vi "Close.vi"(8 "error in":errorcluster, 11 "Cfg Dev in":refnum<class "Configurable Device.lvclass">) -> (0 "error out":errorcluster, 3 "Cfg Dev out":refnum<class "Configurable Device.lvclass">)   [LabVIEW 2018, in "Configurable Device.lvclass"]
uses:
  Configurable Device.lvclass
  Reusable/Session APIs/File Access/Config Data/Config Data.lvclass
  C:/Program Files (x86)/National Instruments/LabVIEW 2018/vi.lib/MSR Consulting, LLC/General Reuse/Session APIs/_Session Fwk/Session - Root.lvclass
  Configurable Device.lvclass/Configurable Device.ctl
  <vilib>/MSR Consulting, LLC/General Reuse/Session APIs/_Session Fwk/Session - Root.lvclass
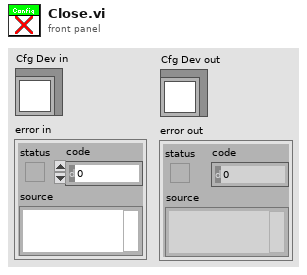
[diagram p1: front panel]
types:
  T1 = typedef "Config Data.lvclass/Config Session.ctl" = refnum<data-value>
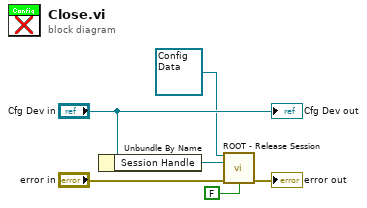
[diagram p0: block diagram]
diagram:
  n1 = Unbundle By Name("Cfg Dev in") -> ("Session Handle"=w4:T1)
  n2 = call <vilib>:"ROOT - Release Session.vi"("OBJ - Session in"=refnum<class "Config Data.lvclass"> refnum ("Config Data"), "Session Handle in"=w4, "error in (no error)"="error in", "force destroy? (F)"=FALSE) -> ("error out"=→"error out":errorcluster)  [unwired: 10 in, 1 out]
  "Cfg Dev out" <- "Cfg Dev in"
